vi "import drone.vi"(10 "drone filepath":path) -> (0 "error out":errorcluster, 2 "Drone":T1)   [LabVIEW 2009]
uses:
  Drone data.ctl
  <vilib>/Utility/config.llb/Read Key (String).vi
  <vilib>/Utility/config.llb/Read Key (I32).vi
  <vilib>/Utility/config.llb/NI_LVConfig.lvlib
  <vilib>/Utility/error.llb/whitespace.ctl
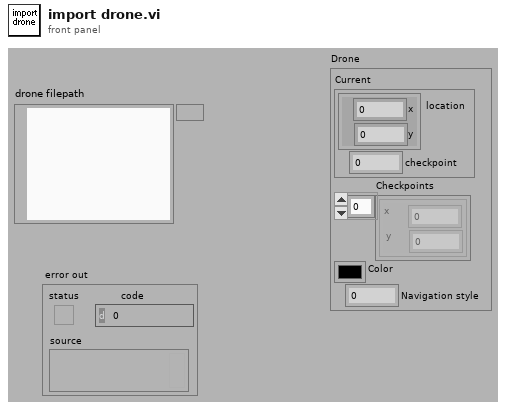
[diagram p1: front panel]
types:
  T1 = typedef "Drone data.ctl" = cluster{"Current":cluster{"location":cluster{"x":i16, "y":i16}, "checkpoint":i32}, "Checkpoints":cluster{"x":i16, "y":i16}[], "Color":u32, "Navigation style":i32}
  T2 = typedef "NI_LVConfig.lvlib/Config Data RefNum.ctl" = refnum<k1>
  T3 = cluster{"default value 1":i32, "default value 1":i32}
  T4 = typedef "whitespace.ctl" = u16
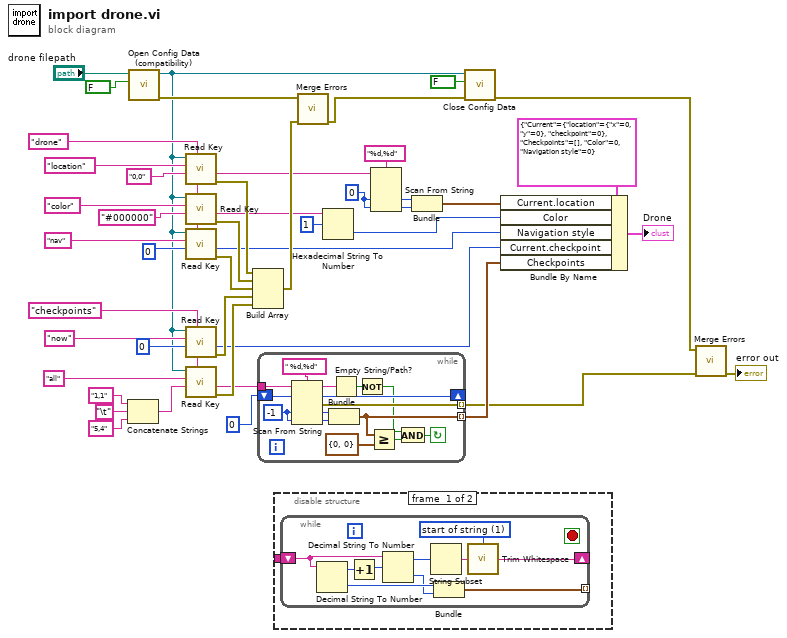
[diagram p0: block diagram]
diagram:
  w8 = i16 0
  w44 = "checkpoints" ("section")
  w40 = "drone" ("section")
  n1 = Concatenate Strings("1,1", "\t", "5,4") -> (w30:string)
  n2 = call <vilib>:"Open Config Data (compatibility).vi"("create file if necessary (T)"=FALSE ("create file if necessary? (T)"), "configuration file path"="drone filepath") -> ("error out"=w21:errorcluster, "refnum"=w5:T2)  [unwired: 7 in, 1 out]
  n3 = call-poly <vilib>:"Read Key.vi"("section"=w40, "default value"="0,0", "key"="location", "refnum"=w5) -> ("error out"=w26:errorcluster, "value"=w9:string)  [unwired: 4 in, 2 out]
  n4 = call-poly <vilib>:"Read Key.vi"("section"=w40, "default value"="#000000", "key"="color", "refnum"=w5) -> ("error out"=w25:errorcluster, "value"=w19:string)  [unwired: 4 in, 2 out]
  n5 = call-poly <vilib>:"Read Key.vi"("section"=w40, "default value"=0, "key"="nav", "refnum"=w5) -> ("error out"=w24:errorcluster, "value"=w16:i32)  [unwired: 4 in, 2 out]
  n6 = call-poly <vilib>:"Read Key.vi"("section"=w44, "default value"=0, "key"="now", "refnum"=w5) -> ("error out"=w23:errorcluster, "value"=w15:i32)  [unwired: 4 in, 2 out]
  n7 = call-poly <vilib>:"Read Key.vi"("section"=w44, "default value"=w30, "key"="all", "refnum"=w5) -> ("error out"=w27:errorcluster, "value"=w14:string)  [unwired: 4 in, 2 out]
  n8 = Build Array(w26, w25, w24, w23, w27) -> (w22:errorcluster[])
  n9 = while {
    tunnel: w14 -> [w58]
    tunnel: [w56] -> w7 mode=indexing
    shift-right: [w53] -> _
    shift-left: u32 0 ("offset past scan") -> [w54]
    tunnel: [w52] -> w2 mode=indexing
    stop <- w48 continue-if-true
    w57 = -1 ("default value 1")
    n10 = Scan From String(format string=" %d,%d", input string=w58, initial scan location=w54, default 1=w57, default 2=w57) -> (remaining string=w51:string, offset past scan=w53:u32, error out=w52:errorcluster, output 1=w60:i32, output 2=w59:i32)  [unwired: 1 in]
    n11 = Bundle("default value 1"=w60, "default value 1"=w59) -> (w56:T3)  [unwired: 1 in]
    n12 = Empty String/Path?(string/path=w51) -> (empty?=w50:bool)
    n13 = Not(x=w50) -> (.not. x?=w47:bool)
    n14 = Greater Or Equal?(x=w56, y=T3 {"default value 1"=0, "default value 1"=0}) -> (x >= y?=w49:bool)
    n15 = And(x=w47, y=w49) -> (x .and. y?=w48:bool)
  }
  n16 = disable-structure shown="Enabled" {
    disable-tunnel: _ -> [w62 _]
    frame #0 {
      n17 = while {
        shift-right: [w67] -> _
        shift-left: w62 -> [w66]
        tunnel: [w63] -> _ mode=indexing
        stop <- _ stop-if-true
        w72 = T4 1 items=["both", "start of string", "end of string"] ("location (both)")
        n18 = Decimal String To Number(string=w66) -> (offset past number=w70:i32, number=w65:i32)  [unwired: 2 in]
        n19 = Increment(x=w70) -> (x+1=w71:i32)
        n20 = Decimal String To Number(string=w66, offset=w71) -> (offset past number=w69:i32, number=w64:i32)  [unwired: 1 in]
        n21 = String Subset(offset (0)=w69) -> (substring=w68:string)  [unwired: 2 in]
        n22 = Bundle(w65, w64) -> (w63:cluster{i32, i32})  [unwired: 1 in]
        n23 = call <vilib>:"Trim Whitespace.vi"("string"=w68, "location (both)"=w72) -> ("trimmed string"=w67:string)
      }
    }
    frame #1 {
    }
  }
  n24 = call <vilib>:"Merge Errors.vi"("error array in"=w22, "error in 1 (no error)"=w21) -> ("error out"=w29:errorcluster)  [unwired: 5 in]
  n25 = Hexadecimal String To Number(string=w19, offset=1) -> (number=w17:u32)  [unwired: 1 in, 1 out]
  n26 = Scan From String(format string="%d,%d", input string=w9, default 1=w8, default 2=w8) -> (output 1=w12:i16, output 2=w13:i16)  [unwired: 2 in, 3 out]
  n27 = Bundle(w12, w13) -> (w10:cluster{i16, i16})  [unwired: 1 in]
  n28 = call <vilib>:"Close Config Data.vi"("error in (no error)"=w29, "write file if changed (T)"=FALSE ("write configuration file? (T)"), "refnum"=w5) -> ("error out"=w3:errorcluster)  [unwired: 7 in, 1 out]
  n29 = Bundle By Name(cluster=T1 {"Current"={"location"={"x"=0, "y"=0}, "checkpoint"=0}, "Checkpoints"=[], "Color"=0, "Navigation style"=0} ("Drone"), "Current.location"=w10, "Color"=w17, "Navigation style"=w16, "Current.checkpoint"=w15, "Checkpoints"=w7) -> (→"Drone":T1)
  n30 = call <vilib>:"Merge Errors.vi"("error array in"=w2, "error in 1 (no error)"=w3) -> ("error out"=→"error out":errorcluster)  [unwired: 5 in]
